vi "第2題.vi"() -> ()   [LabVIEW 2017]
uses:
  <vilib>/Utility/file.llb/Read Delimited Spreadsheet (DBL).vi
  <vilib>/Analysis/NI_AALPro.lvlib
  <vilib>/gmath/NI_Gmath.lvlib
panel:
  out "相關係數":dbl format="%.7g"
  out "all rows":dbl[][](array[numeric])
  out "slope":dbl
  out "appended array":dbl[][](array[numeric])
  in  "file path (dialog if empty)":path
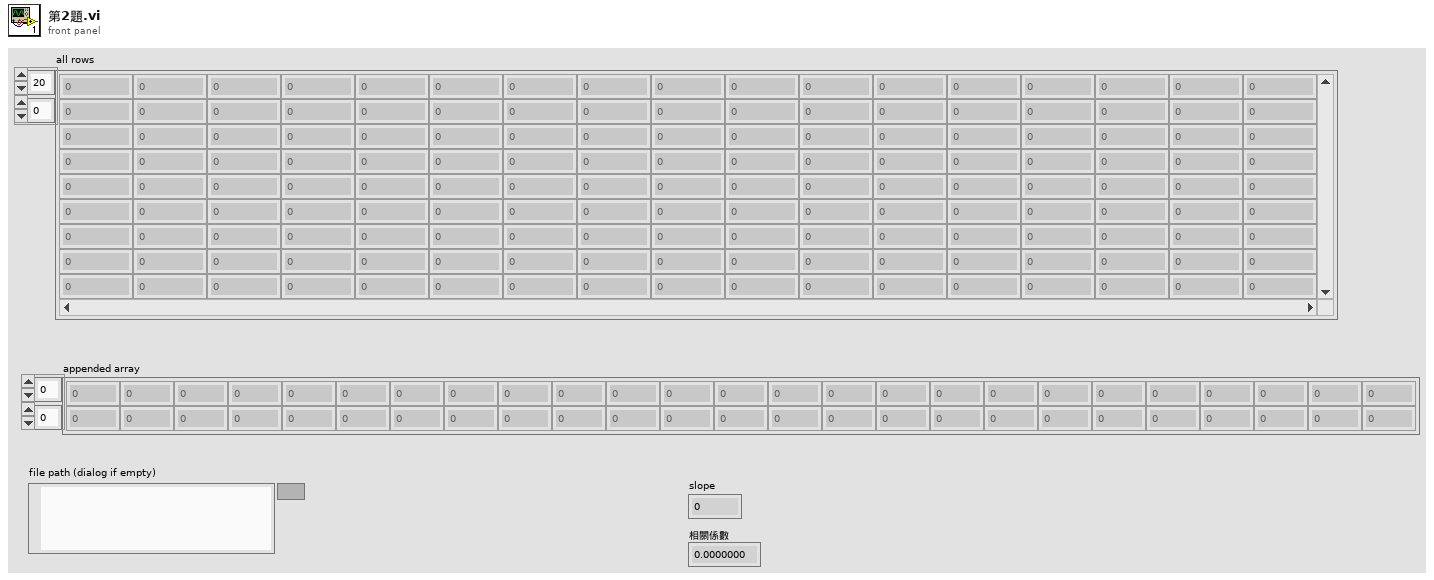
[diagram p1: front panel]
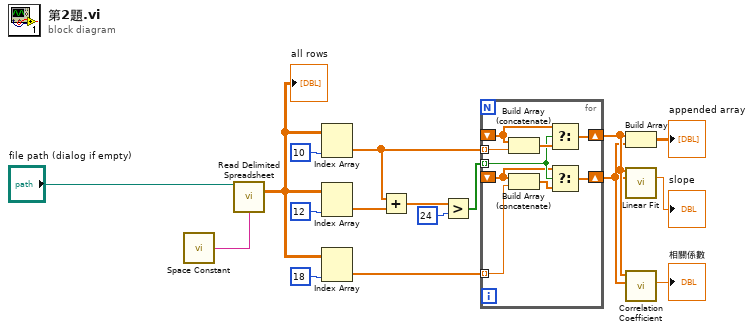
[diagram p0: block diagram]
diagram:
  n1 = call <vilib>:"Space Constant.vi"() -> ("String"=w16:string)
  n2 = call-poly <vilib>:"Read Delimited Spreadsheet.vi"("file path (dialog if empty)"="file path (dialog if empty)", "delimiter (\\t)"=w16) -> ("all rows"=w13:dbl[][])  [unwired: 8 in, 5 out]
  "all rows" <- w13
  n3 = Index Array(array=w13, index (col)=10) -> (element=w7:dbl[])  [unwired: 1 in]
  n4 = Index Array(array=w13, index (col)=12) -> (element=w11:dbl[])  [unwired: 1 in]
  n5 = Index Array(array=w13, index (col)=18) -> (element=w6:dbl[])  [unwired: 1 in]
  n6 = Add(x=w7, y=w11) -> (x+y=w10:dbl[])
  n7 = Greater?(x=w10, y=24) -> (0:w8:bool[])
  n8 = for {
    tunnel: w8 -> [w19] mode=indexing
    tunnel: w7 -> [w26] mode=indexing
    shift-right: [w25] -> w3
    shift-left: _ -> [w23]
    tunnel: w6 -> [w21] mode=indexing
    shift-right: [w20] -> w2
    shift-left: _ -> [w18]
    n9 = Build Array (concatenate)(w23, w26) -> (w24:dbl[])
    n10 = Build Array (concatenate)(w18, w21) -> (w22:dbl[])
    n11 = Select(t=w23, s=w19, f=w24) -> (s? t:f=w25:dbl[])
    n12 = Select(t=w18, s=w19, f=w22) -> (s? t:f=w20:dbl[])
  }
  n13 = Build Array(w3, w2) -> (→"appended array":dbl[][])
  n14 = call <vilib>:"Linear Fit.vi"("Y"=w3, "X"=w2) -> ("slope"=→"slope":dbl)  [unwired: 9 in, 4 out]
  n15 = call <vilib>:"Correlation Coefficient.vi"("Y"=w2, "X"=w3) -> ("r^2"=→"相關係數":dbl)  [unwired: 8 in, 1 out]
